vi "ScpChSetEnabled.vi"(8 "error in (no error)":errorcluster, 9 "Enable?":bool, 10 "wCh in":u16, 11 "hDevice in":u32) -> (0 "error out":errorcluster, 1 "Enabled?":bool, 2 "wCh out":u16, 3 "hDevice out":u32)   [LabVIEW 2018, in "LibTiePie.lvlib"]
uses:
  LibTiePie.lvlib
  LabViewHS4/libtiepie.dll
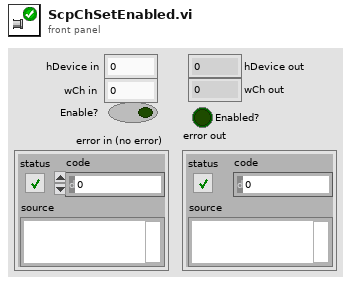
[diagram p1: front panel]
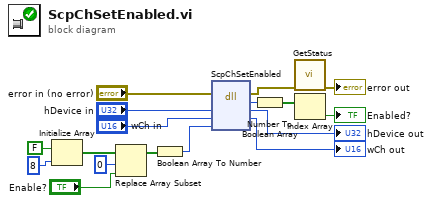
[diagram p0: block diagram]
diagram:
  n1 = Initialize Array(FALSE, 8) -> (w14:bool[])
  n2 = Replace Array Subset(array=w14, new element="Enable?", index=0) -> (w10:bool[])
  n3 = Boolean Array To Number(Boolean array=w10) -> (number=w9:u8)
  n4 = dll-call lib="C:/Users/cwaha/Documents/LabViewHS4/libtiepie.dll" fn="ScpChSetEnabled"(error in="error in (no error)", "hDevice"="hDevice in", "wCh"="wCh in", "bEnable"=w9) -> (error out=w2:errorcluster, "bEnable"=w5:u8, "hDevice"=→"hDevice out":u32, "wCh"=→"wCh out":u16)  [unwired: 3 in, 1 out]
  n5 = Number To Boolean Array(number=w5) -> (Boolean array=w4:bool[])
  n6 = call "GetStatus.vi"("error in (no error)"=w2) -> ("error out"=→"error out":errorcluster)  [unwired: 10 in]
  n7 = Index Array(array=w4) -> (element=→"Enabled?":bool)  [unwired: 1 in]
